vi "get channels.vi"(11 "Polynomial Scale configuration in":refnum<class "Polynomial Scale configuration.lvclass">) -> (2 "channels":refnum<class "TBM channel.lvclass">[](array[class]), 3 "Polynomial Scale configuration out":refnum<class "Polynomial Scale configuration.lvclass">)   [LabVIEW 2013]
uses:
  <vilib>/NI/Tag Bus Module Framework/channel/TBM channel.lvclass
  Polynomial Scale configuration.lvclass
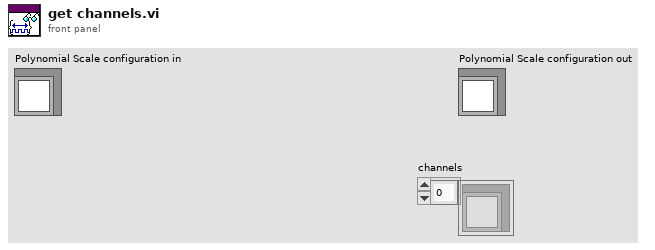
[diagram p1: front panel]
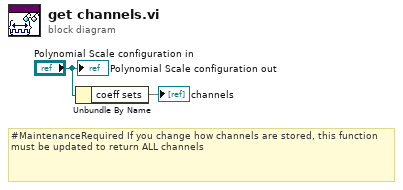
[diagram p0: block diagram]
diagram:
  # "#MaintenanceRequired If you change how channels are stored, this function must be updated to return ALL channels"
  n1 = Unbundle By Name("Polynomial Scale configuration in") -> ("coeff sets"=→"channels")
  "Polynomial Scale configuration out" <- "Polynomial Scale configuration in"
